vi "PlusKey.vi"(8 "error in (no error)":errorcluster caption="错误输入（无错误）") -> (0 "error out":errorcluster caption="错误输出", 1 "布尔":bool, 2 "子字符串":string, 3 "读取缓冲区":string)   [LabVIEW 2018]
uses:
  Subvi/Global.vi
panel:
  in  "字符串 2":string
  in  "停止":bool
  in  "字符串":string
  out "子字符串之后":string
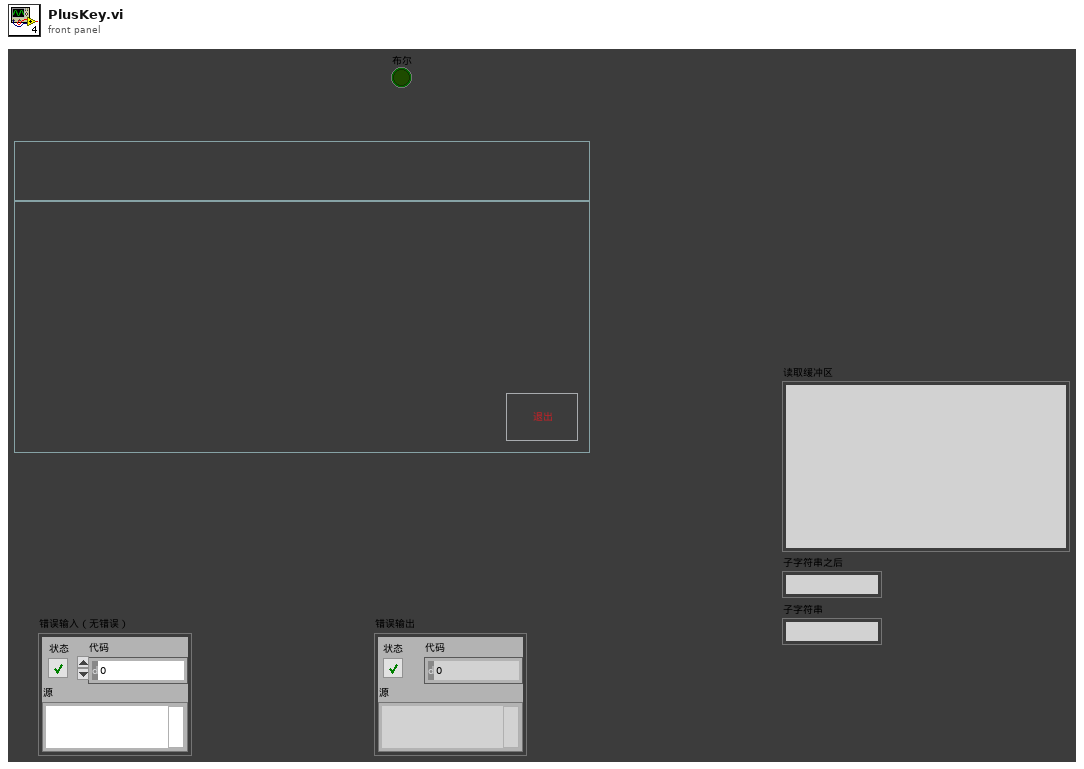
[diagram p1: front panel]
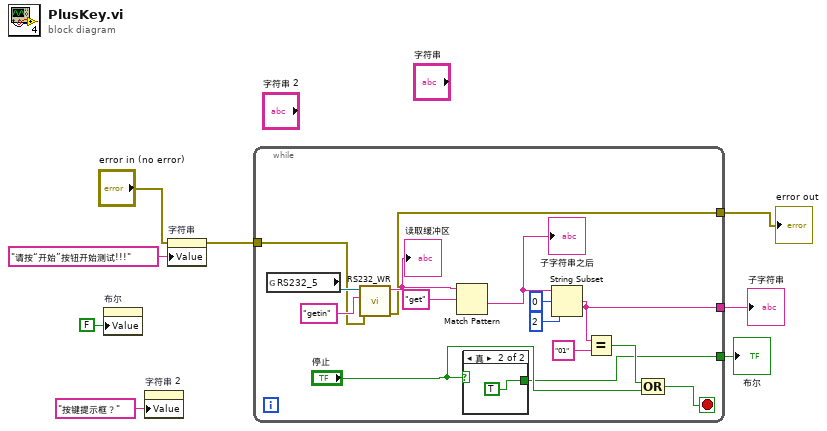
[diagram p0: block diagram]
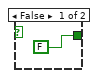
[diagram p2: hidden frame]
diagram:
  n1 = property on="布尔" class="Bool (严格)"("Value"=FALSE ("布尔")) -> ()  [unwired: 2 in, 2 out]
  n2 = property on="字符串 2" class="Str"("Value"="按键提示框？" ("字符串 2")) -> ()  [unwired: 2 in, 2 out]
  n3 = property on="字符串" class="Str"(error in="error in (no error)", "Value"="请按“开始”按钮开始测试!!!" ("字符串")) -> (error out=w7:errorcluster)  [unwired: 1 in, 1 out]
  n4 = while {
    tunnel: [w16] -> w8
    tunnel: w7 -> [w13]
    tunnel: [w14] -> w4
    tunnel: [w9] -> w3
    stop <- w11 stop-if-true
    n5 = global read "Global.vi" "RS232_5"() -> (w23:refnum<visa-resource-name>)
    n6 = call "RS232_WR.vi"("error in (no error)"=w13, "CMD"="getin", "VISA资源名称"=w23) -> ("error out"=w14:errorcluster, "读取缓冲区"=w20:string)  [unwired: 6 in, 1 out]
    "读取缓冲区" <- w20
    n7 = Match Pattern(string=w20, regular expression="get" ("正则表达式")) -> (after substring=w19:string)  [unwired: 1 in, 3 out]
    "子字符串之后" <- w19
    n8 = case shown="真" "停止" {
      tunnel: [FALSE TRUE] -> w9
      frame False {
      }
      frame True {
      }
    }
    n9 = String Subset(string=w19, offset (0)=0 ("偏移量(0)"), length (rest)=2 ("长度（剩余）")) -> (substring=w16:string)
    n10 = Equal?(x=w16, y="01") -> (x = y?=w12:bool)
    n11 = Compound Arithmetic op=OR ("复合运算")(w12, "停止") -> (w11:bool)
  }
  "子字符串" <- w8
  "error out" <- w4
  "布尔" <- w3
